vi "Wait.vi"(0 "Data Task in":refnum<k21>, 5 "data task error in":errorcluster, 7 "#DAQ outputs (1-13)":i32, 9 "PS VISA in":refnum<visa-resource-name>, 11 "PS error in":errorcluster caption="PS error in (no error)", 12 "Wait Filepath":path=path "C:/Users/ga11/Desktop/VI/results/3PtestChrgRest.lvm" caption="Filename", 13 "Wait time":dbl) -> (4 "data task out":refnum<k21>, 6 "data task error out":errorcluster, 10 "PS Visa Out":refnum<visa-resource-name>, 15 "PS error out":errorcluster)   [LabVIEW 2020]
uses:
  Drivers-NHR-9200/NHR/Public/Data/Low Level/Fetch (Ave Voltage).vi
  Drivers-NHR-9200/NHR/NH Research Regenerative Test Series.lvlib
panel:
  out "Ave Current (A)":dbl
  out "Ave Voltage (V)":dbl
  out "WaitElapsed Time (s)":i32 caption="Elapsed Time (s)"
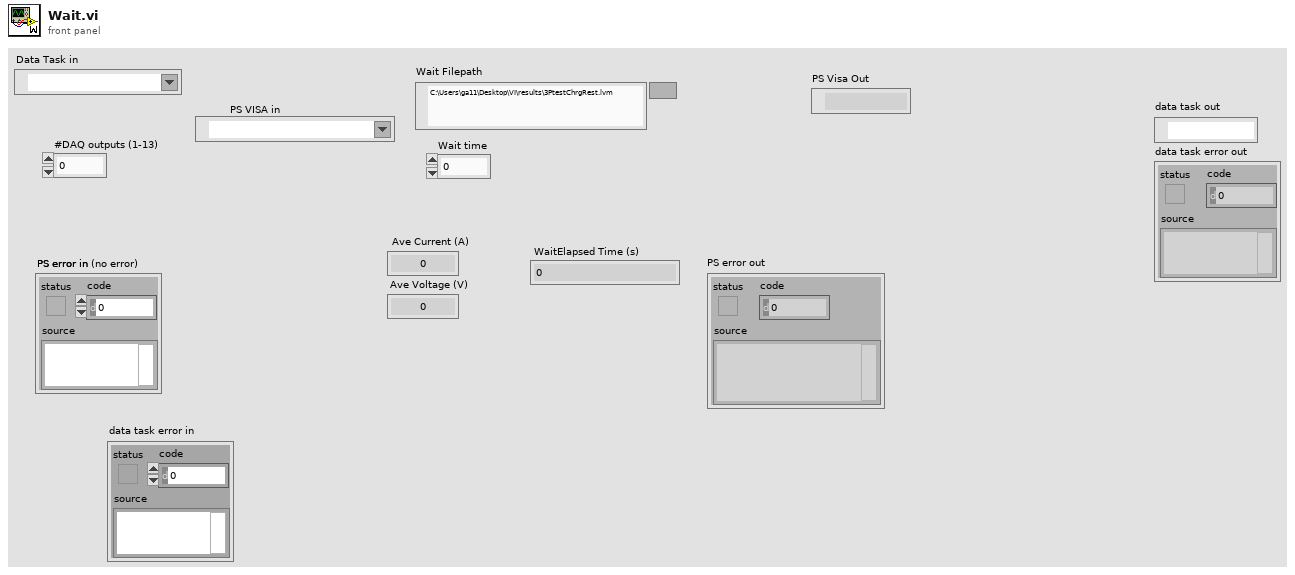
[diagram p1: front panel]
types:
  T1 = cluster{"Voltage Enabled":bool, "Current Enabled":bool, "Power Enabled":bool, "Resistance Enabled":bool}
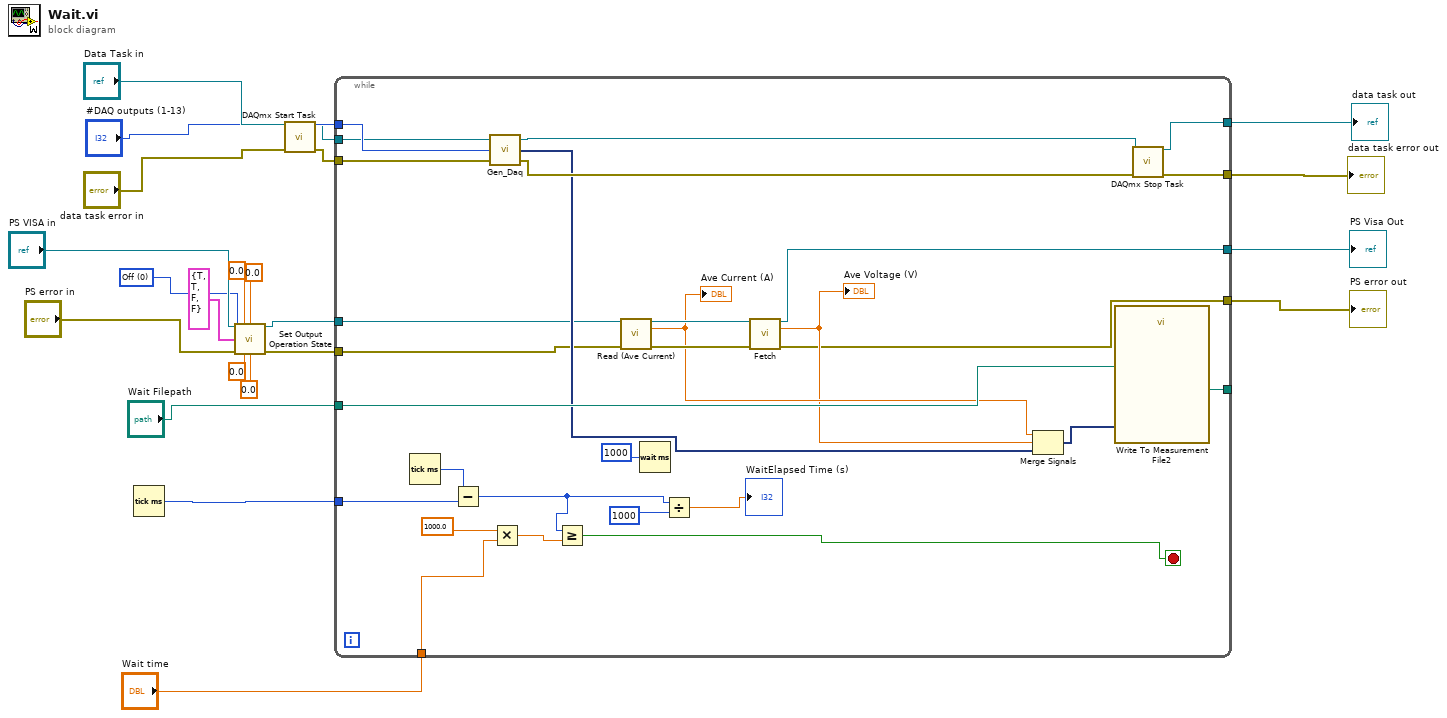
[diagram p0: block diagram]
diagram:
  w8 = 0 items=["Off", "Standby", "Charge", "Discharge", "Battery"] ("Mode (0: Off)")
  n1 = Tick Count (ms)() -> (millisecond timer value=w21:u32)
  n2 = call "Set Output Operation State.vi"("VISA resource name"="PS VISA in", "Voltage Setpoint (0 V)"=0.0, "Current Setpoint (0 A)"=0.0, "Mode (0: Off)"=w8, "Enable"=T1 {"Voltage Enabled"=TRUE, "Current Enabled"=TRUE, "Power Enabled"=FALSE, "Resistance Enabled"=FALSE}, "error in (no error)"="PS error in", "Power Setpoint (0 W)"=0.0, "Resistance Setpoint (0 Ohms)"=0.0) -> ("VISA resource name out"=w9:refnum<visa-resource-name>, "error out"=w5:errorcluster)  [unwired: 6 in]
  n3 = call <vilib>:"DAQmx Start Task.vi"("task/channels in"="Data Task in", "error in"="data task error in") -> ("task out"=w12:refnum<k21>, "error out"=w11:errorcluster)  [unwired: 12 in]
  n4 = while {
    tunnel: "Wait time" -> [w46]
    tunnel: [w43] -> _
    tunnel: w21 -> [w42]
    tunnel: "Wait Filepath" -> [w41]
    tunnel: [w35] -> w19
    tunnel: [w34] -> w18
    tunnel: "#DAQ outputs (1-13)" -> [w31]
    tunnel: w12 -> [w30]
    tunnel: w11 -> [w29]
    tunnel: [w28] -> w14
    tunnel: [w27] -> w13
    tunnel: w9 -> [w24]
    tunnel: w5 -> [w23]
    stop <- w47 stop-if-true
    n5 = Tick Count (ms)() -> (millisecond timer value=w48:u32)
    n6 = Subtract(x=w48, y=w42) -> (x-y=w25:u32)
    n7 = call "Gen_Daq.vi"("error in"=w29, "#DAQ outputs (1-13)"=w31, "task/channels in"=w30) -> ("error out"=w32:errorcluster, "DaQ_output"=w26:dynamicdata, "task out"=w33:refnum<k21>)
    n8 = Multiply(x=1000.0, y=w46) -> (x*y=w44:dbl)
    n9 = Greater Or Equal?(x=w25, y=w44) -> (x >= y?=w47:bool)
    n10 = call "Read (Ave Current).vi"("VISA resource name"=w24, "error in (no error)"=w23) -> ("VISA resource name out"=w50:refnum<visa-resource-name>, "Ave Current (A)"=w38:dbl, "error out"=w51:errorcluster)  [unwired: 11 in]
    "Ave Current (A)" <- w38
    n11 = Wait (ms)(milliseconds to wait=1000) -> ()  [unwired: 1 out]
    n12 = Divide(x=w25, y=1000) -> (x/y=→"WaitElapsed Time (s)":dbl)
    n13 = call-poly "Fetch.vi"("VISA resource name"=w50, "error in (no error)"=w51) -> ("VISA resource name out"=w35:refnum<visa-resource-name>, "Ave Voltage (V)"=w36:dbl, "error out"=w34:errorcluster)  [unwired: 11 in]
    "Ave Voltage (V)" <- w36
    n14 = Merge Signals "Merge Signals"(w38, w36, w26) -> (w37:dynamicdata)
    n15 = call "Write To Measurement File2"("Signals"=w37, "Filename"=w41) -> ("Filename Out"=w43:path)  [unwired: 15 in, 2 out]
    n16 = call <vilib>:"DAQmx Stop Task.vi"("task/channels in"=w33, "error in"=w32) -> ("task out"=w28:refnum<k21>, "error out"=w27:errorcluster)  [unwired: 12 in]
  }
  "PS Visa Out" <- w19
  "PS error out" <- w18
  "data task out" <- w14
  "data task error out" <- w13
